vi "Advance past next JSON Scaler.vi"(7 "JSON":string, 9 "Offset":i32, 11 "State":T1=enum."Leading Whitespace") -> (1 "index":i32, 2 "Value start":i32, 3 "Enum":T1=enum."Undefined")   [LabVIEW 2013, in "JSON2.lvlib"]
uses:
  JSON2.lvlib
  JSON Value Search.ctl
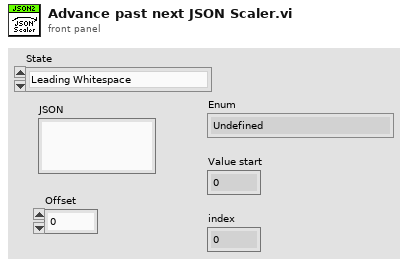
[diagram p1: front panel]
types:
  T1 = typedef "JSON2.lvlib/JSON Value Search.ctl" = enum16{"Parser Error", "In Object", "In Array", "String", "Number", "Leading Whitespace", "Object end", "Array end", "Value end", "Undefined"}
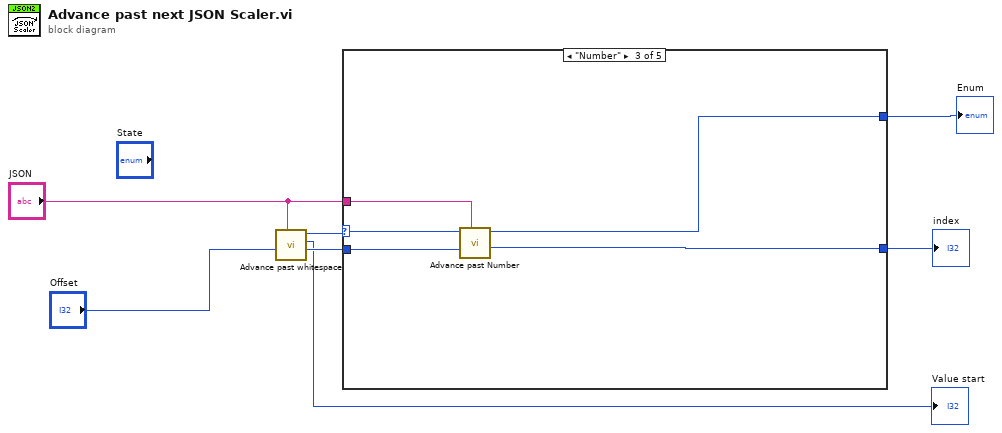
[diagram p0: block diagram]
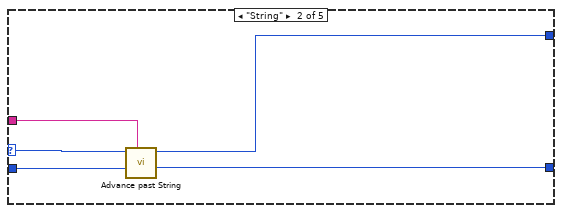
[diagram p3: hidden frame]
diagram:
  n1 = call "Advance past whitespace.vi"("JSON"="JSON", "Offset"="Offset") -> ("Offset past match"=w4:i32, "Offset of first non-whitspace"=→"Value start":i32, "State"=w6:T1)  [unwired: 7 in]
  n2 = case shown="\"Number\"" w6 {
    selector: w6 -> [w8 w13 w18 w21 w22]
    tunnel: "JSON" -> [_ w14 w19 _ _]
    tunnel: w4 -> [w9 w12 w17 w20 w23]
    tunnel: [w9 w11 w16 w20 w23] -> w5
    tunnel: [w8 w10 w15 w21 w22] -> w2
    frame "Parser Error", Default {
    }
    frame "String" {
      n3 = call "Advance past String.vi"("JSON"=w14, "Offset"=w12, "State in"=w13) -> ("Offset past match"=w11:i32, "State"=w10:T1)  [unwired: 6 in, 1 out]
    }
    frame "Number" {
      n4 = call "Advance past Number.vi"("JSON"=w19, "Offset (0)"=w17, "Enum in"=w18) -> ("Offset past match"=w16:i32, "Enum out"=w15:T1)  [unwired: 6 in, 1 out]
    }
    frame "In Object", "In Array" {
      # "Note that big JSON text will have lots of scalers compared to Objects/Arrays"
      # "This VI is inlined, for speed.  We cannot inline anything in a recursive cycle\nso we can't do Arrays/Objects here (must call a non-inlined VI after)"
    }
    frame "Value end" {
      # "null, true, etc."
    }
  }
  "Enum" <- w2
  "index" <- w5
